vi "oooooldand_upload.vi"() -> ()   [LabVIEW 2016]
uses:
  <userlib>/LevyLab/Graph Utilities/graph_utilities.lvclass
  <userlib>/LevyLab/LV to ITX/Data/Data.lvclass
  <userlib>/LevyLab/postgreSQL-timescaleDB/Data.S3/Data.S3.lvclass
  <userlib>/LevyLab/postgreSQL-timescaleDB/Data.PG/Data.PGSQL.lvclass
  <userlib>/LevyLab/Graph Utilities/graph_utilities.lvclass/graph_utilities.ctl
  <userlib>/LevyLab/LV to ITX/Data/Typedefs/File Type--enum.ctl
  <userlib>/LevyLab/LV to ITX/Data/Data.lvclass/Data.ctl
  <userlib>/_OpenG.lib/file/file.llb/File Exists - Scalar__ogtk.vi
  <userlib>/_OpenG.lib/file/file.llb/Build Path - File Names Array__ogtk.vi
  <userlib>/LevyLab/LV to ITX/Macros/Conversion.lvclass
panel:
  out "Intensity Graph":dbl[][](graph)
  out "Notes":string
  out "cache file out":path
  out "Vertical Linecut":cluster{"Array":dbl[], "A x Vector":dbl[]}[](graph) caption="XY Graph"
  out "Horizontal Linecut":cluster{"Array":dbl[], "A x Vector":dbl[]}[](graph) caption="XY Graph"
  in  "# std deviations for\nhistogram width":dbl(slide)=1.4340101522842639 scale=0.0..5.0
  out "Histogram Graph":T1(graph)={"X Values"=[-4.260453721936876e-06, -4.186170219584622e-06, -4.111886717232367e-06, -4.037603214880112e-06, -3.9633197125278575e-06, -3.889036210175604e-06, -3.814752707823349e-06, -3.7404692054710943e-06, -3.6661857031188396e-06, -3.591902200766585e-06, -3.5176186984143303e-06, -3.4433351960620756e-06, -3.369051693709821e-06, -3.294768191357566e-06, -3.2204846890053115e-06, -3.1462011866530572e-06, -3.0719176843008025e-06, -2.9976341819485483e-06, -2.9233506795962936e-06, -2.849067177244039e-06, -2.774783674891784e-06, -2.7005001725395295e-06, -2.626216670187275e-06, -2.55193316783502e-06, -2.4776496654827654e-06, -2.4033661631305107e-06, -2.3290826607782565e-06, -2.2547991584260018e-06, -2.180515656073747e-06, -2.106232153721493e-06, -2.031948651369238e-06, -1.9576651490169834e-06, -1.8833816466647288e-06, -1.809098144312474e-06, -1.7348146419602196e-06, -1.6605311396079651e-06, -1.5862476372557104e-06, -1.5119641349034557e-06, -1.437680632551201e-06, -1.3633971301989466e-06, -1.289113627846692e-06, -1.2148301254944374e-06, -1.1405466231421827e-06, -1.066263120789928e-06, -9.919796184376733e-07, -9.176961160854188e-07, -8.434126137331644e-07, -7.691291113809097e-07, -6.94845609028655e-07, -6.205621066764003e-07, -5.462786043241458e-07, -4.7199510197189133e-07, -3.9771159961963664e-07, -3.2342809726738195e-07, -2.4914459491512726e-07, -1.7486109256287257e-07, -1.0057759021061788e-07, -2.6294087858363186e-08, 4.798941449389108e-08, 1.2227291684614535e-07, 1.9655641919840004e-07, 2.7083992155065473e-07, 3.451234239029094e-07, 4.194069262551641e-07, 4.936904286074188e-07, 5.679739309596735e-07, 6.422574333119282e-07, 7.165409356641829e-07, 7.908244380164376e-07, 8.651079403686918e-07, 9.393914427209461e-07, 1.0136749450732008e-06, 1.0879584474254555e-06, 1.1622419497777102e-06, 1.2365254521299649e-06, 1.3108089544822195e-06, 1.3850924568344742e-06, 1.459375959186729e-06, 1.5336594615389836e-06, 1.6079429638912379e-06, 1.6822264662434922e-06, 1.7565099685957468e-06, 1.8307934709480015e-06, 1.9050769733002562e-06, 1.979360475652511e-06, 2.0536439780047656e-06, 2.1279274803570203e-06, 2.202210982709275e-06, 2.2764944850615297e-06, 2.3507779874137844e-06, 2.4250614897660386e-06, 2.499344992118293e-06, 2.5736284944705476e-06, 2.6479119968228023e-06, 2.722195499175057e-06, 2.7964790015273117e-06, 2.8707625038795664e-06, 2.945046006231821e-06, 3.0193295085840757e-06, 3.09361301093633e-06], "Histogram: h(x)"=[55, 64, 64, 55, 89, 72, 77, 95, 93, 93, 89, 83, 103, 107, 94, 103, 104, 123, 108, 131, 122, 143, 132, 148, 168, 174, 204, 248, 183, 187, 243, 200, 217, 226, 238, 254, 185, 182, 212, 219, 221, 318, 385, 545, 593, 736, 735, 784, 778, 858, 957, 1241, 1705, 2411, 3715, 13259, 21719, 20305, 20447, 22279, 10136, 3576, 2142, 1564, 1112, 936, 844, 776, 734, 696, 601, 535, 390, 337, 334, 301, 271, 341, 294, 279, 254, 216, 170, 148, 122, 140, 100, 114, 127, 147, 102, 114, 129, 135, 110, 105, 90, 91, 93, 96]}
  in  "menu select":T2(tab)
  in  "Populate Local Tree":bool
  in  "Local Tree":string(tree)
  in  "S3 Connect":bool
  in  "local data directory":path=path "C:/bigdata/PPMS2/SA03008N.20190801/031_sg1_-1'1''5m_3AC=500m_bg=-14" caption="Path"
  in  "Load":bool
  in  "Regen Cache":bool
  out "generating cache":bool
  out "reading cache":bool
  out "cache found":bool
  in  "Visualize":bool
  out "itx load (ms)":u32
  out "cache load (ms)":u32
  out "generate cache (ms)":u32
  out "data dimensions":i32[](array[numeric])
  in  "Remote Tree":string(tree)
  in  "Button":bool
  in  "object path for AWS download":string
  in  "Download\nfrom AWS":bool
  in  "Upload\nto AWS":bool
  out "TDMS file exists on AWS":bool
  out "downloaded file":path
  in  "aws bucket":string="levylab-data"
  in  "path to aws credentials":path=path "C:/Users/phil/.aws/credentials"
  in  "connection info":T3
  in  "Add Op":bool
  in  "Operations List":i32(listbox)
  in  "update":bool
  out "updating":bool
  in  "auto\nupdate":bool
  in  "trash can":i32(listbox)
  in  "OK":bool
  # "4"
  # "7"
  # "10"
  # "12"
  # "14"
  # "Settings"
  # "17"
  # "(e.g. SA03008N.20190801)"
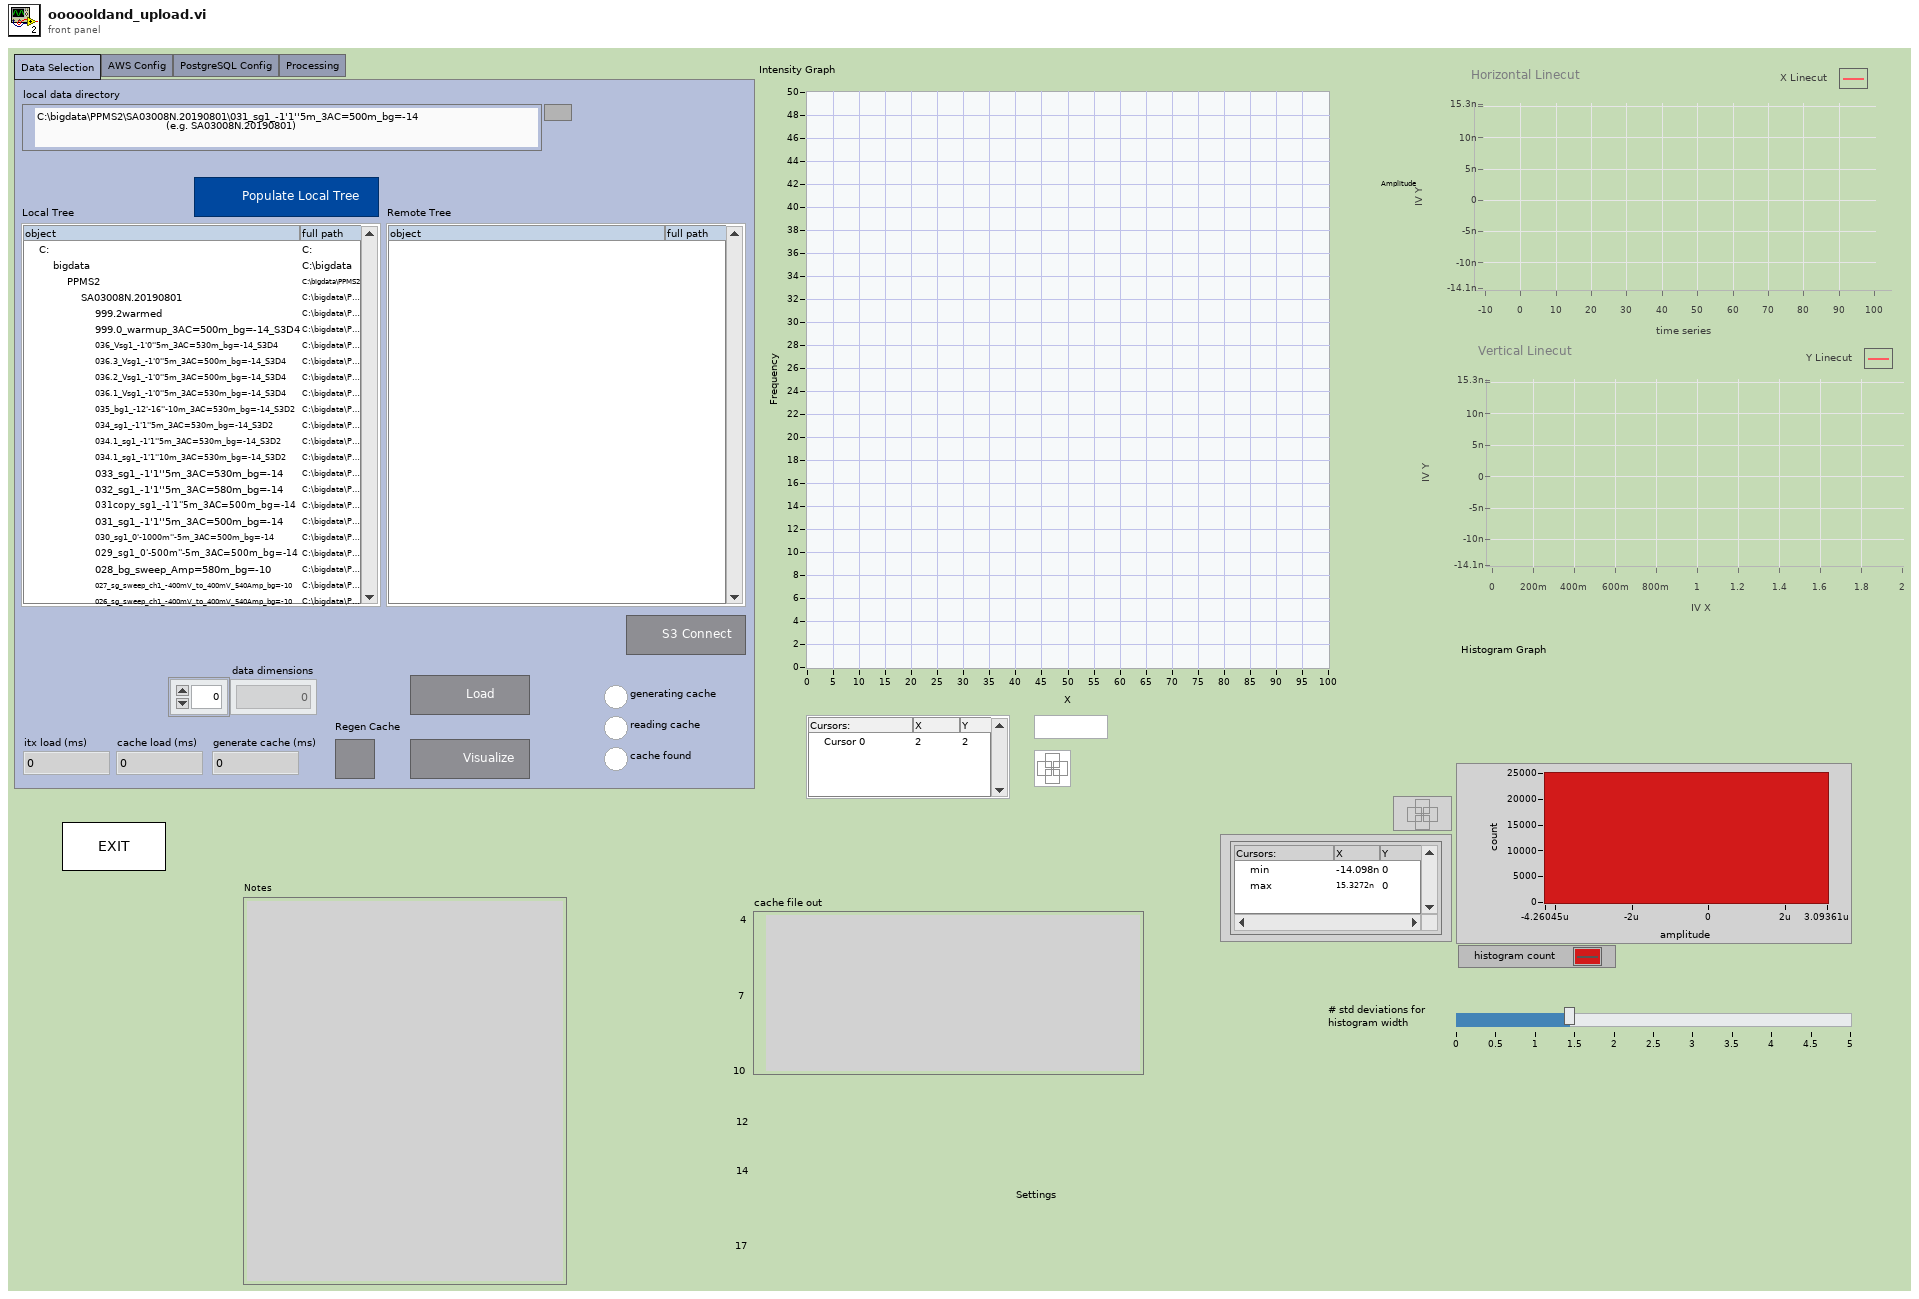
[diagram p1: front panel]
types:
  T1 = cluster{"X Values":dbl[], "Histogram: h(x)":i32[]}
  T2 = enum32{"Data Selection", "AWS Config", "PostgreSQL Config", "Processing"}
  T3 = cluster{"host":string, "port":string, "user":string, "dbname":string, "password":string}
  T4 = enum32{"Invalid", "Standard", "Closed", "Hidden", "Minimized", "Maximized"}
  T5 = enum32{"invalid app kind", "Development System", "Run Time System", "Student Edition", "Embedded LabVIEW", "Evaluation", "Custom"}
  T6 = typedef "Data.lvclass/File Type--enum.ctl" = enum16{"DAT", "ITX", "TDMS", "VI"}
  T7 = typedef "Dictionary Object RefNum__ogtk.ctl" = refnum<k1>
  T8 = cluster{"Core":cluster{"Current VI Reference":refnum<vi>, "Close Panel on Exit?":bool}, "active XY data":cluster{"All expt data":dbl[], "All expt data":dbl[]}[], "local data directory":path, "Data Save":refnum<class "Data.lvclass">, "graphs":refnum<class "graph_utilities.lvclass">[], "dictionary out":T7, "Operations List":refnum<vi>, "operations performed":string[], "Histogram Data":cluster{"X Values":dbl[], "Histogram: h(x)":i32[]}, "Histogram Graph":refnum<vi>, "wavenames":string[], "Data.S3":refnum<class "Data.S3.lvclass">, "data dimensions":i32[], "Data.PG in":refnum<class "Data.PGSQL.lvclass">}
  T9 = cluster{"All expt data":dbl[], "All expt data":dbl[]}[]
  T10 = cluster{"Current VI Reference":refnum<vi>, "Close Panel on Exit?":bool}
  T11 = typedef "Data.lvclass/Dictionary--cluster.ctl" = cluster{"key":string, "value":variant}
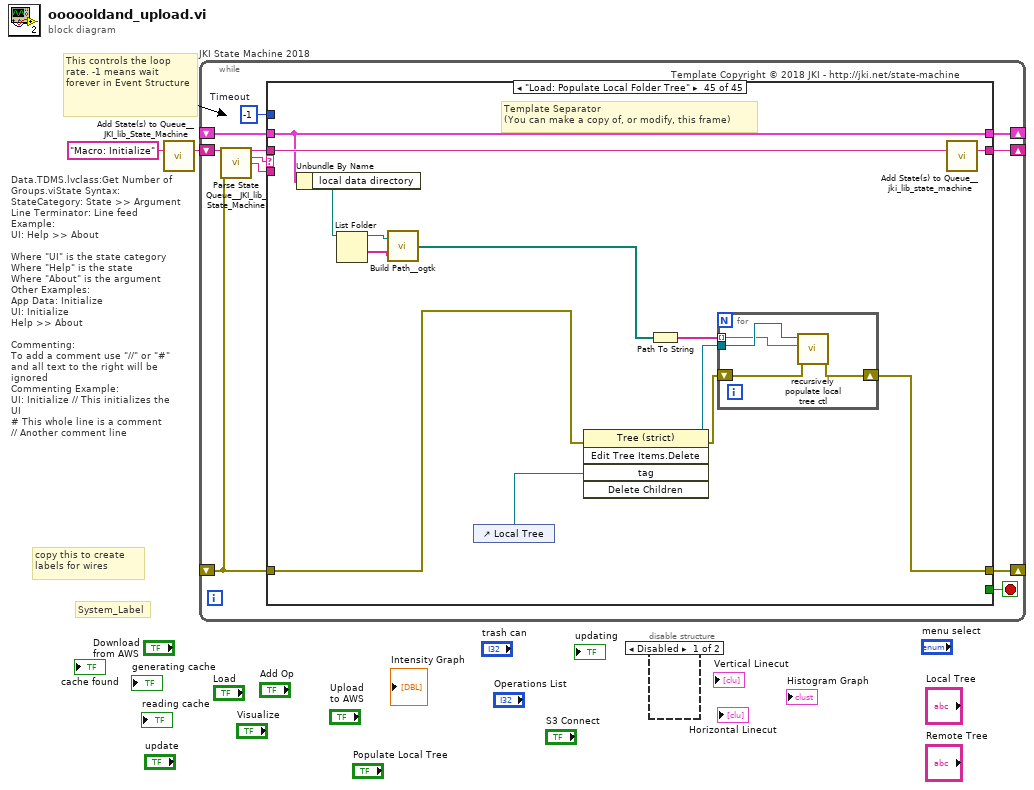
[diagram p0: block diagram]
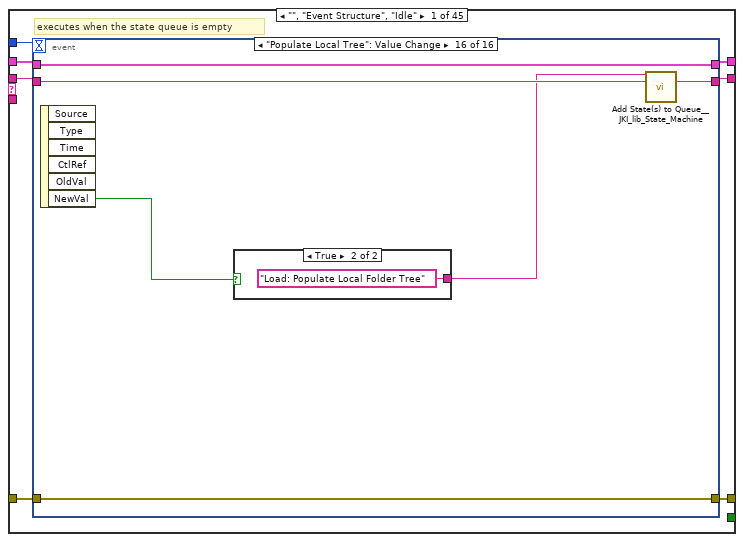
[diagram p3: hidden frame]
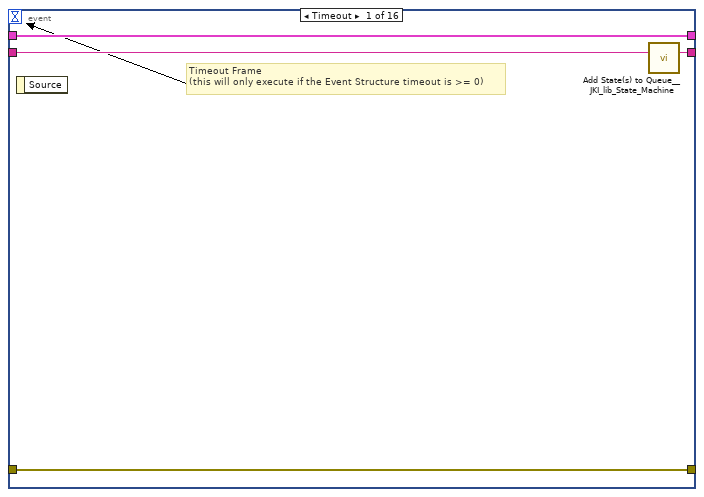
[diagram p4: hidden frame]
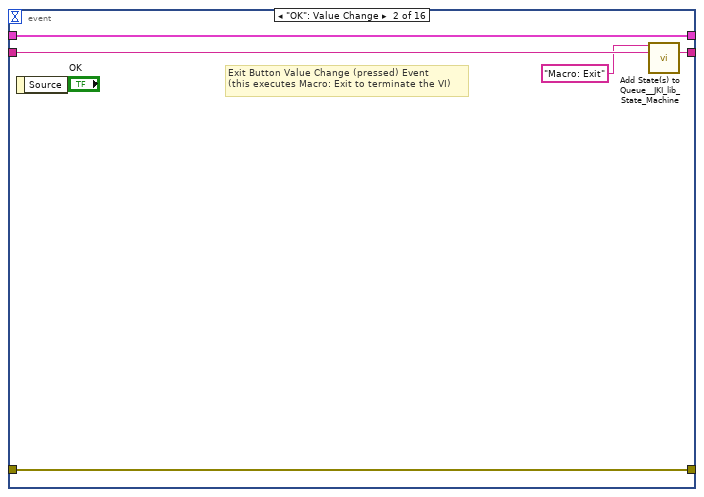
[diagram p5: hidden frame]
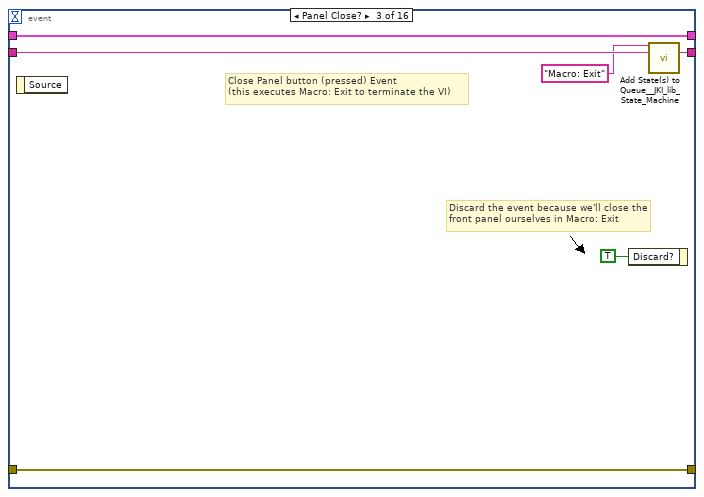
[diagram p6: hidden frame]
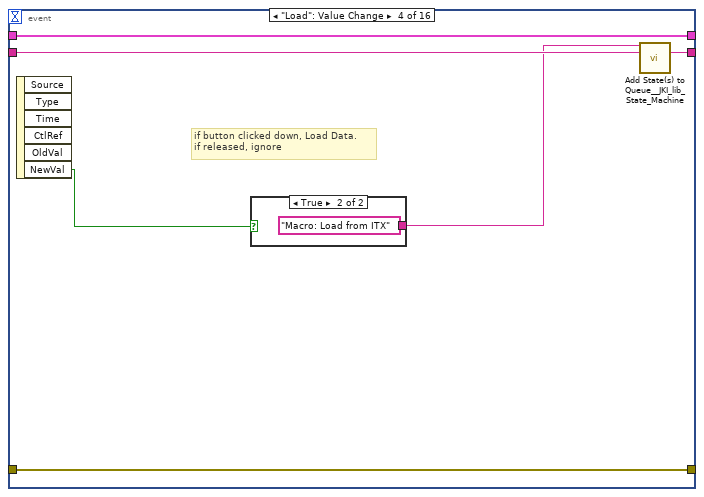
[diagram p7: hidden frame]
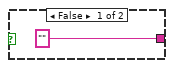
[diagram p8: hidden frame]
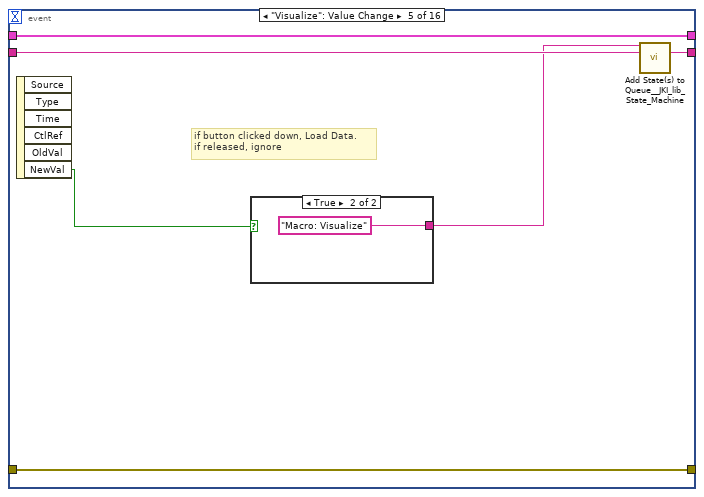
[diagram p9: hidden frame]
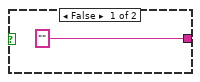
[diagram p10: hidden frame]
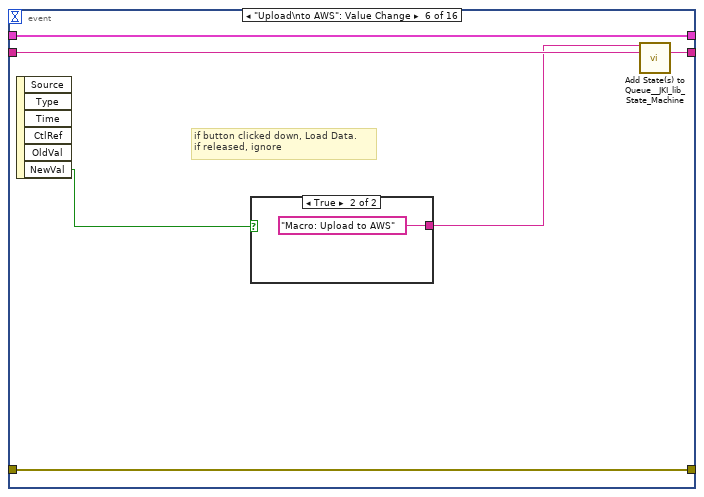
[diagram p11: hidden frame]
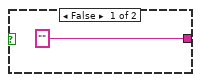
[diagram p12: hidden frame]
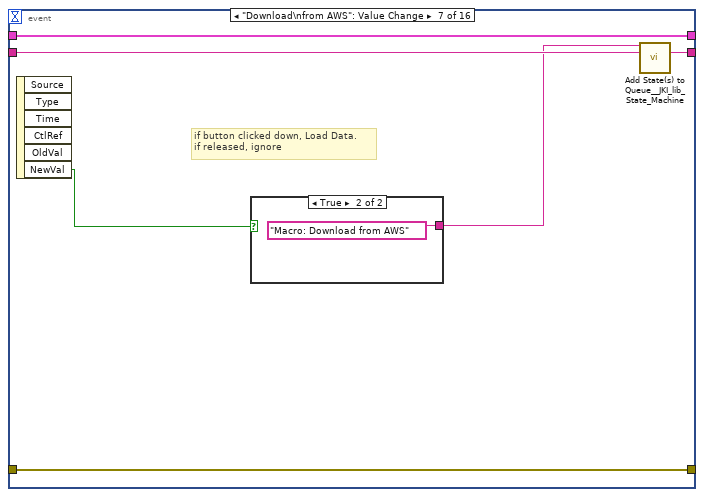
[diagram p13: hidden frame]
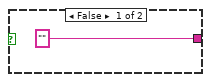
[diagram p14: hidden frame]
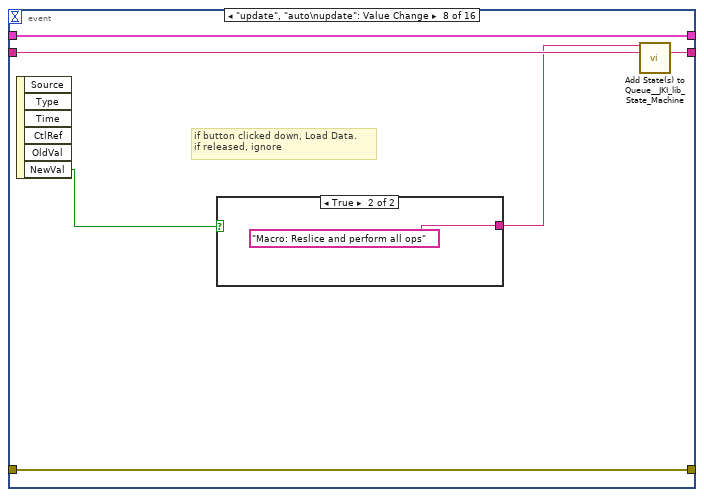
[diagram p15: hidden frame]
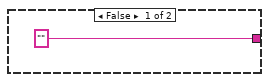
[diagram p16: hidden frame]
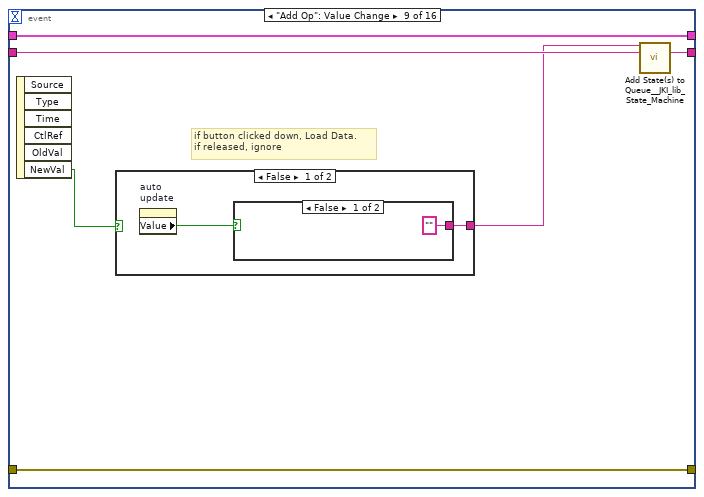
[diagram p17: hidden frame]
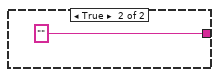
[diagram p18: hidden frame]
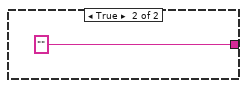
[diagram p19: hidden frame]
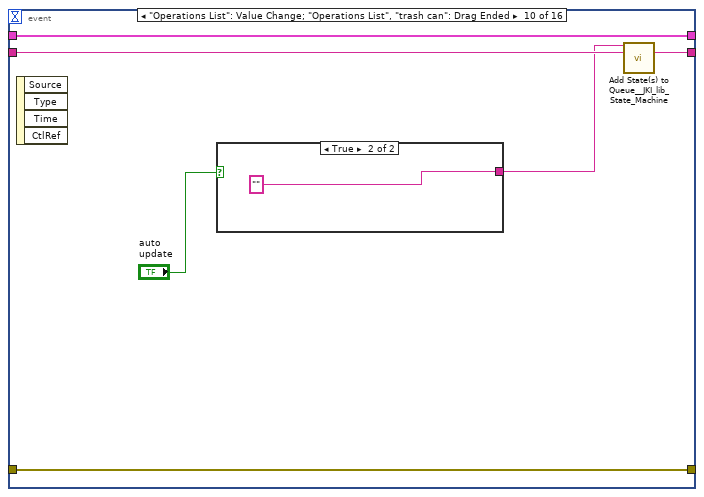
[diagram p20: hidden frame]
diagram:
  # "Data.TDMS.lvclass:Get Number of Groups.viState Syntax:\nStateCategory: State >> Argument\nLine Terminator: Line feed\nExample:\nUI: Help >> About\n\nWhere \"UI\" is the state category\nWhere \"Help\" is the state\nWhere \"About\" is the argument\nOther Examples:\nApp Data: Initialize\nUI: Initialize\nHelp >> About\n\nCommenting:\nTo add a comment use \"//\" or \"#\" and all text to the right will be ignored\nCommenting Example:\nUI: Initialize // This initializes the UI\n# This whole line is a comment\n// Another comment line"
  # "copy this to create labels for wires"
  # "This controls the loop rate. -1 means wait forever in Event Structure"
  # "System_Label"
  n1 = call <vilib>:"Add State(s) to Queue__JKI_lib_State_Machine.vi"("State(s) in (\"\")"="Macro: Initialize") -> ("States Out"=w2:string)  [unwired: 14 in]
  n2 = while "JKI State Machine 2018" {
    shift-right: [w6] -> _
    shift-left: _ -> [w3]
    shift-right: [w9] -> _
    shift-left: _ -> [w4]
    shift-right: [w8] -> _
    shift-left: w2 -> [w10]
    stop <- w7 stop-if-true
    w5 = -1  # Timeout
    # "Template Copyright © 2018 JKI - http://jki.net/state-machine"
    n3 = call <vilib>:"Parse State Queue__JKI_lib_State_Machine.vi"("State Queue"=w10, "Error In (no error)"=w4) -> ("Remaining States"=w12:string, "Current State"=w13:string, "Arguments"=w11:string)  [unwired: 11 in]
    n4 = case shown="\"Load: Populate Local Folder Tree\"" w13 {
      selector: w13 -> [_ _ w137 _ _ _ _ _ _ _ _ _ _ _ _ _ _ _ _ _ _ _ _ _ _ _ _ _ _ _ _ _ _ _ _ _ _ _ _ _ _ _ _ _ _]
      tunnel: w12 -> [w20 w136 w141 w160 w166 w171 w175 w196 w220 w226 w230 w234 w240 w251 w320 w325 w330 w335 w340 w345 w350 w355 w365 w369 w373 w377 w381 w394 w408 w431 w454 w458 w463 w467 w471 w484 w499 w517 w531 w535 w556 w585 w618 w630 w646]
      tunnel: w11 -> [_ _ _ _ _ _ _ _ _ _ _ _ w235 w245 _ _ _ _ _ _ _ _ _ _ _ _ _ _ _ _ _ _ _ _ _ _ _ _ _ _ _ _ _ _ _]
      tunnel: w3 -> [w18 w133 w139 w153 w163 w169 w172 _ w208 w221 w227 w232 w238 w247 w317 w322 w327 w332 w337 w342 w347 w352 w362 w366 w370 w374 w378 w392 w397 w410 w452 w455 w460 w464 w468 w476 w495 w515 w529 w532 w537 w577 w611 w627 w634]
      tunnel: [w17 w134 w143 w157 errorcluster {"status"=FALSE, "code"=0, "source"=""} ("error out") w168 w173 w189 w214 w222 w228 w231 w236 w248 w318 w323 w326 w331 w336 w341 w346 w351 w363 w367 w371 w375 w379 w387 w398 w421 w447 w456 w461 w465 w469 w474 w487 w508 w521 w533 w546 w580 w613 w622 w641] -> w9
      tunnel: w4 -> [w16 w134 w142 w157 w162 w168 w173 w190 w198 w223 w228 w231 w237 w249 w318 w323 w326 w331 w336 w341 w346 w351 w363 w367 w371 w375 w379 w388 w399 w415 w441 w456 w461 w465 w469 w477 w496 w509 w522 w533 w548 w579 w615 w625 w636]
      tunnel: [w19 w135 w140 w159 w165 w170 w174 w195 w219 w225 w229 w233 w239 w250 w319 w324 w329 w334 w339 w344 w349 w354 w364 w368 w372 w376 w380 w393 w407 w430 w453 w457 w462 w466 w470 w483 w498 w516 w530 w534 w555 w584 w617 w629 w645] -> w8
      tunnel: [_ _ _ _ _ TRUE _ _ _ _ _ _ _ _ _ _ _ _ _ _ _ _ _ _ _ _ _ _ _ _ _ _ _ _ _ _ _ _ _ _ _ _ _ _ _] -> w7
      tunnel: [w15 w133 w139 w158 w163 w169 w172 w194 w218 w221 w227 w232 w238 w247 w317 w322 w327 w332 w337 w342 w347 w352 w362 w366 w370 w374 w378 w392 w396 w411 w452 w455 w460 w464 w468 w476 w495 w515 w529 w532 w537 w577 w610 w628 w634] -> w6
      tunnel: w5 -> [w14 _ _ _ _ _ _ _ _ _ _ _ _ _ _ _ _ _ _ _ _ _ _ _ _ _ _ _ _ _ _ _ _ _ _ _ _ _ _ _ _ _ _ _ _]
      frame "", "Event Structure", "Idle" {
        # "executes when the state queue is empty"
        n5 = event shown="[15] \"Populate Local Tree\": Value Change" {
          selector: _ -> [_ _ _ _ _ _ _ _ _ _ _ _ _ _ _ _]
          dyn-events: _ -> [_ _ _ _ _ _ _ _ _ _ _ _ _ _ _ _]
          timeout: w14 -> [_ _ _ _ _ _ _ _ _ _ _ _ _ _ _ _]
          tunnel: w20 -> [w24 w29 w35 w38 w46 w54 w62 w70 w78 w91 w96 w104 w109 w113 w119 w127]
          tunnel: [w23 w28 w34 w39 w47 w55 w63 w71 w79 w90 w97 w103 w108 w114 w120 w128] -> w19
          tunnel: w18 -> [w21 w26 w32 w41 w49 w57 w65 w73 w81 w87 w100 w106 w111 w116 w122 w130]
          tunnel: [w22 w27 w33 w40 w48 w56 w64 w72 w80 w92 w101 w105 w110 w115 w121 w129] -> w17
          tunnel: w16 -> [w22 w27 w33 w40 w48 w56 w64 w72 w80 w92 w101 w105 w110 w115 w121 w129]
          tunnel: [w21 w26 w32 w41 w49 w57 w65 w73 w81 w87 w99 w106 w111 w116 w122 w130] -> w15
          event Timeout {
            # "Timeout Frame\n(this will only execute if the Event Structure timeout is >= 0)"
            n6 = event-data() -> ()  [unwired: 1 in, 1 out]
            n7 = call <vilib>:"Add State(s) to Queue__JKI_lib_State_Machine.vi"("State(s) in (\"\")"=w24) -> ("States Out"=w23:string)  [unwired: 14 in]
          }
          event "OK": Value Change {
            # "Exit Button Value Change (pressed) Event\n(this executes Macro: Exit to terminate the VI)"
            n8 = event-data() -> ()  [unwired: 1 in, 1 out]
            n9 = call <vilib>:"Add State(s) to Queue__JKI_lib_State_Machine.vi"("State(s) in Front (\"\")"="Macro: Exit", "State(s) in (\"\")"=w29) -> ("States Out"=w28:string)  [unwired: 13 in]
          }
          event Panel Close? {
            # "Discard the event because we'll close the front panel ourselves in Macro: Exit"
            # "Close Panel button (pressed) Event\n(this executes Macro: Exit to terminate the VI)"
            n10 = event-data() -> ()  [unwired: 1 in, 1 out]
            n11 = event-data("Discard?"=TRUE) -> ()  [unwired: 1 in, 1 out]
            n12 = call <vilib>:"Add State(s) to Queue__JKI_lib_State_Machine.vi"("State(s) in Front (\"\")"="Macro: Exit", "State(s) in (\"\")"=w35) -> ("States Out"=w34:string)  [unwired: 13 in]
          }
          event "Load": Value Change {
            # "if button clicked down, Load Data.\nif released, ignore"
            n13 = event-data() -> ("NewVal"=w37:bool)  [unwired: 1 in, 5 out]
            n14 = case shown="True" w37 {
              tunnel: ["" "Macro: Load from ITX"] -> w36
              frame False {
              }
              frame True {
              }
            }
            n15 = call <vilib>:"Add State(s) to Queue__JKI_lib_State_Machine.vi"("State(s) in Front (\"\")"=w36, "State(s) in (\"\")"=w38) -> ("States Out"=w39:string)  [unwired: 13 in]
          }
          event "Visualize": Value Change {
            # "if button clicked down, Load Data.\nif released, ignore"
            n16 = event-data() -> ("NewVal"=w45:bool)  [unwired: 1 in, 5 out]
            n17 = case shown="True" w45 {
              tunnel: ["" "Macro: Visualize"] -> w44
              frame False {
              }
              frame True {
              }
            }
            n18 = call <vilib>:"Add State(s) to Queue__JKI_lib_State_Machine.vi"("State(s) in Front (\"\")"=w44, "State(s) in (\"\")"=w46) -> ("States Out"=w47:string)  [unwired: 13 in]
          }
          event "Upload\nto AWS": Value Change {
            # "if button clicked down, Load Data.\nif released, ignore"
            n19 = event-data() -> ("NewVal"=w53:bool)  [unwired: 1 in, 5 out]
            n20 = case shown="True" w53 {
              tunnel: ["" "Macro: Upload to AWS"] -> w52
              frame False {
              }
              frame True {
              }
            }
            n21 = call <vilib>:"Add State(s) to Queue__JKI_lib_State_Machine.vi"("State(s) in Front (\"\")"=w52, "State(s) in (\"\")"=w54) -> ("States Out"=w55:string)  [unwired: 13 in]
          }
          event "Download\nfrom AWS": Value Change {
            # "if button clicked down, Load Data.\nif released, ignore"
            n22 = event-data() -> ("NewVal"=w61:bool)  [unwired: 1 in, 5 out]
            n23 = case shown="True" w61 {
              tunnel: ["" "Macro: Download from AWS"] -> w60
              frame False {
              }
              frame True {
              }
            }
            n24 = call <vilib>:"Add State(s) to Queue__JKI_lib_State_Machine.vi"("State(s) in Front (\"\")"=w60, "State(s) in (\"\")"=w62) -> ("States Out"=w63:string)  [unwired: 13 in]
          }
          event "update", "auto\nupdate": Value Change {
            # "if button clicked down, Load Data.\nif released, ignore"
            n25 = event-data() -> ("NewVal"=w69:bool)  [unwired: 1 in, 5 out]
            n26 = case shown="True" w69 {
              tunnel: ["" "Macro: Reslice and perform all ops"] -> w68
              frame False {
              }
              frame True {
              }
            }
            n27 = call <vilib>:"Add State(s) to Queue__JKI_lib_State_Machine.vi"("State(s) in Front (\"\")"=w68, "State(s) in (\"\")"=w70) -> ("States Out"=w71:string)  [unwired: 13 in]
          }
          event "Add Op": Value Change {
            # "if button clicked down, Load Data.\nif released, ignore"
            n28 = event-data() -> ("NewVal"=w77:bool)  [unwired: 1 in, 5 out]
            n29 = case shown="False" w77 {
              tunnel: [w83 ""] -> w76
              frame False {
                n30 = property on="auto\nupdate" class="Bool (strict)"() -> ("Value"=w82:bool)  [unwired: 2 in, 2 out]
                n31 = case shown="False" w82 {
                  tunnel: ["" ""] -> w83
                  frame False {
                  }
                  frame True {
                  }
                }
              }
              frame True {
              }
            }
            n32 = call <vilib>:"Add State(s) to Queue__JKI_lib_State_Machine.vi"("State(s) in Front (\"\")"=w76, "State(s) in (\"\")"=w78) -> ("States Out"=w79:string)  [unwired: 13 in]
          }
          event "Operations List": Value Change; "Operations List", "trash can": Drag Ended {
            n33 = event-data() -> ()  [unwired: 1 in, 4 out]
            n34 = case shown="True" "auto\nupdate" {
              tunnel: ["" ""] -> w89
              frame False {
              }
              frame True {
              }
            }
            n35 = call <vilib>:"Add State(s) to Queue__JKI_lib_State_Machine.vi"("State(s) in Front (\"\")"=w89, "State(s) in (\"\")"=w91) -> ("States Out"=w90:string)  [unwired: 13 in]
          }
          event "local data directory": Value Change {
            # "if button clicked down, Load Data.\nif released, ignore"
            n36 = event-data() -> ("NewVal"=w95:path)  [unwired: 1 in, 5 out]
            n37 = Bundle By Name(cluster=w100, "local data directory"=w95) -> (w99:T8)
            n38 = call <vilib>:"Add State(s) to Queue__JKI_lib_State_Machine.vi"("State(s) in Front (\"\")"="Load: Check for Cache" ("State(s) in Front (\"\")"), "State(s) in (\"\")"=w96) -> ("States Out"=w97:string)  [unwired: 13 in]
          }
          event "Histogram Graph": Cursor Move {
            n39 = event-data() -> ()  [unwired: 1 in, 9 out]
            n40 = call <vilib>:"Add State(s) to Queue__JKI_lib_State_Machine.vi"("State(s) in Front (\"\")"="Visualize: Update Z from Histogram" ("State(s) in Front (\"\")"), "State(s) in (\"\")"=w104) -> ("States Out"=w103:string)  [unwired: 13 in]
          }
          event "# std deviations for\nhistogram width": Value Change {
            n41 = event-data() -> ()  [unwired: 1 in, 6 out]
            n42 = call <vilib>:"Add State(s) to Queue__JKI_lib_State_Machine.vi"("State(s) in Front (\"\")"="Visualize: Calculate Histogram\nVisualize: Update Z from Histogram" ("State(s) in Front (\"\")"), "State(s) in (\"\")"=w109) -> ("States Out"=w108:string)  [unwired: 13 in]
          }
          event "Intensity Graph": Cursor Move {
            n43 = event-data() -> ()  [unwired: 1 in, 9 out]
            n44 = call <vilib>:"Add State(s) to Queue__JKI_lib_State_Machine.vi"("State(s) in Front (\"\")"="Visualize: Line Cuts" ("State(s) in Front (\"\")"), "State(s) in (\"\")"=w113) -> ("States Out"=w114:string)  [unwired: 13 in]
          }
          event "S3 Connect": Value Change {
            n45 = event-data() -> ("NewVal"=w117:bool)  [unwired: 1 in, 5 out]
            n46 = case shown="True" w117 {
              tunnel: ["" "Macro: Connect to AWS S3" ("State(s) in Front (\"\")")] -> w118
              frame False {
              }
              frame True {
              }
            }
            n47 = call <vilib>:"Add State(s) to Queue__JKI_lib_State_Machine.vi"("State(s) in Front (\"\")"=w118, "State(s) in (\"\")"=w119) -> ("States Out"=w120:string)  [unwired: 13 in]
          }
          event "Populate Local Tree": Value Change {
            n48 = event-data() -> ("NewVal"=w125:bool)  [unwired: 1 in, 5 out]
            n49 = case shown="True" w125 {
              tunnel: ["" "Load: Populate Local Folder Tree" ("State(s) in Front (\"\")")] -> w126
              frame False {
              }
              frame True {
              }
            }
            n50 = call <vilib>:"Add State(s) to Queue__JKI_lib_State_Machine.vi"("State(s) in Front (\"\")"=w126, "State(s) in (\"\")"=w127) -> ("States Out"=w128:string)  [unwired: 13 in]
          }
        }
      }
      frame "---------- Core ----------" {
        # "Do not put any code in this frame.\n(it is a separator no-op)"
        n51 = call <vilib>:"Add State(s) to Queue__jki_lib_state_machine.vi"("State(s) in (\"\")"=w136) -> ("States Out"=w135:string)  [unwired: 14 in]
      }
      frame Default {
        w146 = 42 items=["No error", "Argument error", "Memory is full", "Out of zone", "End of file", "File already open", "Generic file I/O error", "File not found", "File permission error", "Disk is full", "Duplicate path", "Too many files open", "System feature not enabled", "Resource file not found", "Cannot add resource", "Resource not found", "Image not found", "Image memory error", "Pen does not exist", "Config type invalid", "Config token not found", "Config parse error", "Config memory error", "Bad external code format", "Bad external code offset", "External code not present", "Null window", "Destroy window error", "Null menu", "Print aborted", "Bad print record", "Print driver error", "Windows error during printing", "Memory error during printing", "Print dialog error", "Generic print error", "Invalid device refnum", "Device not found", "Device parameter error", "Device unit error", "Cannot open device", "Device call aborted", "Generic error", "Cancelled by user", "Object ID too low", "Object ID too high", "Object not in heap", "Unknown heap", "Unknown object (invalid DefProc)", "Unknown object (DefProc not in table)", "Message out of range", "Invalid (null) method", "Unknown message", "Manager call not supported", "Bad address", "Network operation in progress", "Network operation timed out", "Connection is busy", "Network attribute not supported", "Network error", "Address in use", "System out of memory", "Connection aborted", "Connection refused", "Not connected", "Already connected", "Connection closed", "Initialization error (interapplication manager)", "Bad occurrence", "Wait on unbound occurrence handler", "Occurrence queue overflow", "Datalog type conflict", "Unused", "Unrecognized type (interapplication manager)", "Memory corrupt", "Failed to make temporary DLL", "Old CIN version", "Drag socket not found", "Failed to load drop-object", "Failed to register OLE object", "Failed to release OLE object", "Format specifier type mismatch", "Unknown format specifier", "Too few format specifiers", "Too many format specifiers", "Scan failed", "Newer CIN version", "Error converting to variant", "Runtime menu error", "Password tampered", "Variant attribute not found", "Incompatible variant data type", "Event data is not available", "Event Store is not present", "Occurrence is not found", "Event Queue is not created", "Event info is not available", "Refnum passed is NULL", "Error retrieving Class GUID", "Error retrieving CoClass GUID", "Error retrieving TypeLib GUID.", "Bad built application magic bytes.", "Specific driver is different from the specific driver associated with the Logical Name.", "There is no session opened to the class driver.", "Max Error", "MAX - Error with config objects", "MAX - Error loading configuration", "MAX - Group not supported"]
        # "Current State"
        # "Do not delete, rename, or modify this frame.\n(this is used to capture unhandled states and typos)"
        # "Handle mistyped state name (developer tool)"
        n52 = Format Into String(format string="Software Exception: Unhandled State \"%s\"." ("message"), error in=w142, w137) -> (resulting string=w145:string, error out=w144:errorcluster)  [unwired: 1 in]
        n53 = call <vilib>:"Error Cluster From Error Code.vi"("show call chain? (False)"=TRUE, "error in (no error)"=w144, "error message (\"\")"=w145, "error code (0)"=w146) -> ("error out"=w143:errorcluster)  [unwired: 5 in]
        n54 = call <vilib>:"Add State(s) to Queue__jki_lib_state_machine.vi"("State(s) in (\"\")"=w141) -> ("States Out"=w140:string)  [unwired: 14 in]
      }
      frame "Initialize Core Data" {
        # "Do not delete, rename, or modify this frame.\n(this is used to determine panel behavior on exit)"
        # "originally closed?"
        # "exe?"
        # "If panel starts closed or is an EXE, then close it when we exit"
        n55 = property class="VI"() -> ("FP.State"=w150:T4)  [unwired: 2 in, 2 out]
        n56 = property class="App"() -> ("App.Kind"=w156:T5)  [unwired: 2 in, 2 out]
        n57 = control-ref of="Current VI Reference"() -> (w151:refnum<vi>)
        n58 = Equal?(x=w150, y=T4."Closed" ("Front Panel Window:State")) -> (x = y?=w148:bool)
        n59 = Equal?(x=w156, y=T5."Run Time System" ("Application:Kind")) -> (x = y?=w154:bool)
        n60 = Or(x=w148, y=w154) -> (x .or. y?=w152:bool)
        n61 = Bundle By Name(cluster=w153, "Core.Current VI Reference"=w151, "Core.Close Panel on Exit?"=w152) -> (w158:T8)
        n62 = call <vilib>:"Add State(s) to Queue__jki_lib_state_machine.vi"("State(s) in (\"\")"=w160) -> ("States Out"=w159:string)  [unwired: 14 in]
      }
      frame "Error Handler" {
        # "Unhandled Error -- Display it"
        # "Handle any errors here.\nYou can also output any states to clean-up after errors occur"
        # "Clear error"
        n63 = call <vilib>:"General Error Handler.vi"("error in (no error)"=w162) -> ()  [unwired: 10 in, 5 out]
        n64 = call <vilib>:"Add State(s) to Queue__jki_lib_state_machine.vi"("State(s) in Front (\"\")"="/* Post Error States", "State(s) in (\"\")"=w166) -> ("States Out"=w165:string)  [unwired: 13 in]
      }
      frame "Exit" {
        # "Do not put any code in this frame.\n(No errors that occur here will be handled.)"
        n65 = call <vilib>:"Add State(s) to Queue__jki_lib_state_machine.vi"("State(s) in (\"\")"=w171) -> ("States Out"=w170:string)  [unwired: 14 in]
      }
      frame "---------- Data ----------" {
        # "Do not put any code in this frame.\n(It is a separator no-op. You can make a copy of this frame to create a new Data frame)"
        n66 = call <vilib>:"Add State(s) to Queue__jki_lib_state_machine.vi"("State(s) in (\"\")"=w175) -> ("States Out"=w174:string)  [unwired: 14 in]
      }
      frame "Data: Initialize" {
        w177 = i32[] []  # data dimensions
        w178 = refnum<class "Data.S3.lvclass"> refnum  # Data.S3
        w179 = string[] []  # wavenames
        w183 = T1 {"X Values"=[], "Histogram: h(x)"=[]}  # Histogram Data
        w184 = string[] []  # operations performed
        w186 = T9 []  # active XY data
        w185 = string[] [] ("Strings []")
        w192 = refnum<class "graph_utilities.lvclass">[] []  # graphs
        w193 = T10 {"Current VI Reference"=refnum, "Close Panel on Exit?"=FALSE}  # Core
        # "# groups in tdms\n    (i.e. # original itx files)\n# channels (time, AIN, AON,\n# points per channel\n    (except the channels\n     that only store 1)"
        # "do not delete - used by framework"
        # "Data names and types of shift register data are defined by this bundle."
        # "Initialize the shift-register data, here.\n(data names are defined by what you wire into the bundle function)"
        n67 = call <userlib>:"Dictionary Create__ogtk.vi"("error in (no error)"=w190) -> ("error out"=w189:errorcluster, "dictionary out"=w191:T7)  [unwired: 9 in]
        n68 = control-ref of="Operations List"() -> (w187:refnum<vi>)
        n69 = property on="trash can" class="LstBox (strict)"("Item Names"=w185) -> ()  [unwired: 2 in, 2 out]
        n70 = property class="LstBox (strict)"(reference=w187, "Item Names"=w185) -> (reference out=w188:refnum<vi>)  [unwired: 1 in, 1 out]
        n71 = control-ref of="Histogram Graph"() -> (w182:refnum<vi>)
        n72 = Bundle("Core"=w193, "active XY data"=w186, "local data directory"="local data directory", "Data Save"=refnum<class "Data.lvclass"> refnum, "graphs"=w192, "dictionary out"=w191, "Operations List"=w188, "operations performed"=w184, "Histogram Data"=w183, "Histogram Graph"=w182, "wavenames"=w179, "Data.S3"=w178, "data dimensions"=w177, "Data.PG in"=refnum<class "Data.PGSQL.lvclass"> refnum) -> (w194:T8)  [unwired: 1 in]
        n73 = call <vilib>:"Add State(s) to Queue__jki_lib_state_machine.vi"("State(s) in (\"\")"=w196) -> ("States Out"=w195:string)  [unwired: 14 in]
      }
      frame "Data: Initialize Graph References" {
        # "need to somehow set credentials and bucket"
        n74 = control-ref of="Local Tree"() -> (w201:refnum<vi>)
        n75 = invoke on="Invoke Node" class="Tree (strict)" method="Edit Tree Items.Delete"(reference=w201, error in=w198) -> (error out=w199:errorcluster)  [unwired: 3 in, 4 out]
        n76 = control-ref of="Vertical Linecut"() -> (w211:refnum<vi>)
        n77 = control-ref of="Intensity Graph"() -> (w202:refnum<vi>)
        n78 = Unbundle By Name(w208) -> ("Data.S3"=w207:refnum<class "Data.S3.lvclass">)
        n79 = control-ref of="Remote Tree"() -> (w200:refnum<vi>)
        n80 = control-ref of="Horizontal Linecut"() -> (w212:refnum<vi>)
        n81 = invoke on="Invoke Node" class="Tree (strict)" method="Edit Tree Items.Delete"(reference=w200, error in=w199) -> (error out=w197:errorcluster)  [unwired: 3 in, 4 out]
        n82 = call <userlib>:"Read Credentials from File.vi"("path to aws credentials"="path to aws credentials", "Data.S3"=w207) -> ("Data.S3 out"=w203:refnum<class "Data.S3.lvclass">)  [unwired: 8 in, 1 out]
        n83 = call <userlib>:"Set Bucket.vi"("Bucket name"="aws bucket", "Data.S3"=w203) -> ("Data.S3"=w206:refnum<class "Data.S3.lvclass">)  [unwired: 8 in, 1 out]
        n84 = call <userlib>:"Write Intensity Graph ref.vi"("error in (no error)"=w197, "Intensity Graph (Control)"=w202, "Intensity Graph"=w202) -> ("error out"=w216:errorcluster, "graph_utilities out"=w210:refnum<class "graph_utilities.lvclass">)  [unwired: 7 in]
        n85 = call <userlib>:"Write XY Graph ref.vi"("error in (no error)"=w216, "XY Graph"=w211, "graph_utilities in"=w210) -> ("error out"=w215:errorcluster, "graph_utilities out"=w209:refnum<class "graph_utilities.lvclass">)  [unwired: 7 in]
        n86 = call <userlib>:"Write XY Graph ref.vi"("error in (no error)"=w215, "XY Graph"=w212, "graph_utilities in"=w210) -> ("error out"=w214:errorcluster, "graph_utilities out"=w213:refnum<class "graph_utilities.lvclass">)  [unwired: 7 in]
        n87 = Build Array(w210, w209, w213) -> (w217:refnum<class "graph_utilities.lvclass">[])
        n88 = Bundle By Name(cluster=w208, "graphs"=w217, "Data.S3"=w206) -> (w218:T8)
        n89 = call <vilib>:"Add State(s) to Queue__jki_lib_state_machine.vi"("State(s) in (\"\")"=w220) -> ("States Out"=w219:string)  [unwired: 14 in]
      }
      frame "Data: Cleanup" {
        # "Cleanup any data and references, here.\n(this is called automatically, by the Macro: Exit)"
        n90 = Unbundle By Name(w221) -> ("Core.Current VI Reference"=w224:refnum<vi>)
        n91 = Close Reference(reference=w224, error in (no error)=w223) -> (error out=w222:errorcluster)
        n92 = call <vilib>:"Add State(s) to Queue__jki_lib_state_machine.vi"("State(s) in (\"\")"=w226) -> ("States Out"=w225:string)  [unwired: 14 in]
      }
      frame "---------- UI ----------" {
        # "Do not put any code in this frame.\n(It is a separator no-op. You can make a copy of this frame to create a new UI frame)"
        n93 = call <vilib>:"Add State(s) to Queue__jki_lib_state_machine.vi"("State(s) in (\"\")"=w230) -> ("States Out"=w229:string)  [unwired: 14 in]
      }
      frame "UI: Initialize" {
        # "Initialize the User Interface, here.\n(this is called automatically, by the Macro: Init)"
        n94 = call <vilib>:"Add State(s) to Queue__jki_lib_state_machine.vi"("State(s) in (\"\")"=w234) -> ("States Out"=w233:string)  [unwired: 14 in]
      }
      frame "UI: Cursor Set" {
        # "Argument"
        # "Set and Unset Cursor Busy.\n(Usage: \"UI: Cursor Set >> Busy|Idle\")"
        n95 = case shown="\"Idle\", Default" w235 {
          tunnel: w237 -> [w242 w244]
          tunnel: [w241 w243] -> w236
          frame "Idle", Default {
            n96 = call <vilib>:"Unset Busy.vi"("error in (no error)"=w242) -> ("error out"=w241:errorcluster)  [unwired: 10 in]
          }
          frame "Busy" {
            n97 = call <vilib>:"Set Busy.vi"("error in (no error)"=w244) -> ("error out"=w243:errorcluster)  [unwired: 9 in, 1 out]
          }
        }
        n98 = call <vilib>:"Add State(s) to Queue__jki_lib_state_machine.vi"("State(s) in (\"\")"=w240) -> ("States Out"=w239:string)  [unwired: 14 in]
      }
      frame "UI: Front Panel State" {
        # "Argument"
        # "Set Front Panel Open or Closed\n(Usage: \"UI: Front Panel State >> Open|Close\")"
        n99 = Unbundle By Name(w247) -> ("Core.Current VI Reference"=w246:refnum<vi>)
        n100 = case shown="\"Minimize\", \"Minimized\"" w245 {
          tunnel: w249 -> [w257 w272 w283 w296 w309]
          tunnel: [w259 w273 w285 w298 w311] -> w248
          tunnel: w246 -> [w258 w270 w284 w297 w310]
          frame "Open", "Standard", Default {
            w252 = T4."Standard" ("State")
            n101 = property class="VI"(reference=w258, error in=w257) -> (reference out=w255:refnum<vi>, error out=w256:errorcluster, "FP.State"=w254:T4)
            n102 = Not Equal?(x=w254, y=w252) -> (x != y?=w253:bool)
            n103 = case shown="True" w253 {
              tunnel: [w263 w265] -> w259
              tunnel: w256 -> [w262 w265]
              tunnel: w255 -> [w261 _]
              tunnel: w252 -> [w260 _]
              frame True {
                n104 = invoke class="VI" method="FP.Open"(reference=w261, error in=w262, "Activate"=TRUE, "State"=w260) -> (error out=w263:errorcluster)  [unwired: 1 in, 4 out]
              }
              frame False {
              }
            }
          }
          frame "Close", "Closed" {
            n105 = property class="VI"(reference=w270, error in=w272) -> (reference out=w269:refnum<vi>, error out=w271:errorcluster, "FP.State"=w267:T4)
            n106 = Not Equal?(x=w267, y=T4."Closed" ("Front Panel Window:State")) -> (x != y?=w266:bool)
            n107 = case shown="True" w266 {
              tunnel: [w274 w277] -> w273
              tunnel: w271 -> [w274 w276]
              tunnel: w269 -> [_ w275]
              frame False {
              }
              frame True {
                n108 = invoke class="VI" method="FP.Close"(reference=w275, error in=w276) -> (error out=w277:errorcluster)  [unwired: 1 in, 2 out]
              }
            }
          }
          frame "Hidden", "Hide" {
            w278 = T4."Hidden" ("State")
            n109 = property class="VI"(reference=w284, error in=w283) -> (reference out=w281:refnum<vi>, error out=w282:errorcluster, "FP.State"=w280:T4)
            n110 = Not Equal?(x=w280, y=w278) -> (x != y?=w279:bool)
            n111 = case shown="True" w279 {
              tunnel: [w289 w290] -> w285
              tunnel: w282 -> [w288 w290]
              tunnel: w281 -> [w287 _]
              tunnel: w278 -> [w286 _]
              frame True {
                n112 = invoke class="VI" method="FP.Open"(reference=w287, error in=w288, "State"=w286) -> (error out=w289:errorcluster)  [unwired: 2 in, 4 out]
              }
              frame False {
              }
            }
          }
          frame "Minimize", "Minimized" {
            w291 = T4."Minimized" ("State")
            n113 = property class="VI"(reference=w297, error in=w296) -> (reference out=w294:refnum<vi>, error out=w295:errorcluster, "FP.State"=w293:T4)
            n114 = Not Equal?(x=w293, y=w291) -> (x != y?=w292:bool)
            n115 = case shown="True" w292 {
              tunnel: [w302 w303] -> w298
              tunnel: w295 -> [w301 w303]
              tunnel: w294 -> [w300 _]
              tunnel: w291 -> [w299 _]
              frame True {
                n116 = invoke class="VI" method="FP.Open"(reference=w300, error in=w301, "State"=w299) -> (error out=w302:errorcluster)  [unwired: 2 in, 4 out]
              }
              frame False {
              }
            }
          }
          frame "Maximize", "Maximized" {
            w304 = T4."Maximized" ("State")
            n117 = property class="VI"(reference=w310, error in=w309) -> (reference out=w307:refnum<vi>, error out=w308:errorcluster, "FP.State"=w306:T4)
            n118 = Not Equal?(x=w306, y=w304) -> (x != y?=w305:bool)
            n119 = case shown="True" w305 {
              tunnel: [w315 w316] -> w311
              tunnel: w308 -> [w314 w316]
              tunnel: w307 -> [w313 _]
              tunnel: w304 -> [w312 _]
              frame True {
                n120 = invoke class="VI" method="FP.Open"(reference=w313, error in=w314, "State"=w312) -> (error out=w315:errorcluster)  [unwired: 2 in, 4 out]
              }
              frame False {
              }
            }
          }
        }
        n121 = call <vilib>:"Add State(s) to Queue__jki_lib_state_machine.vi"("State(s) in (\"\")"=w251) -> ("States Out"=w250:string)  [unwired: 14 in]
      }
      frame "---------- Macro ----------" {
        # "Do not put any code in this frame.\n(It is a separator no-op. You can make a copy of this frame to create a new Macro frame)"
        n122 = call <vilib>:"Add State(s) to Queue__jki_lib_state_machine.vi"("State(s) in (\"\")"=w320) -> ("States Out"=w319:string)  [unwired: 14 in]
      }
      frame "Macro: Initialize" {
        w321 = "Data: Initialize\nData: Initialize Graph References\nInitialize Core Data\nUI: Initialize\nUI: Front Panel State >> Open\nLoad: Check for Cache"  # Data: Initialize Data: Initialize Graph References Initialize Core Data UI: Initialize UI: Front Panel State >> Open Load: Check for Cache
        # "Initialization Macro\n(This is called once, when the VI starts)"
        n123 = call <vilib>:"Add State(s) to Queue__jki_lib_state_machine.vi"("State(s) in Front (\"\")"=w321, "State(s) in (\"\")"=w325) -> ("States Out"=w324:string)  [unwired: 13 in]
      }
      frame "Macro: Load from ITX" {
        # "Initialization Macro\n(This is called once, when the VI starts)"
        n124 = call <vilib>:"Add State(s) to Queue__jki_lib_state_machine.vi"("State(s) in Front (\"\")"="Load: Load from ITX", "State(s) in (\"\")"=w330) -> ("States Out"=w329:string)  [unwired: 13 in]
      }
      frame "Macro: Connect to AWS S3" {
        # "Initialization Macro\n(This is called once, when the VI starts)"
        n125 = call <vilib>:"Add State(s) to Queue__jki_lib_state_machine.vi"("State(s) in Front (\"\")"="AWS: List Bucket Contents", "State(s) in (\"\")"=w335) -> ("States Out"=w334:string)  [unwired: 13 in]
      }
      frame "Macro: Visualize" {
        # "#TODO: should rename this macro,\nit only needs to be sliced after the slicing indices are changed"
        # "Initialization Macro\n(This is called once, when the VI starts)"
        n126 = call <vilib>:"Add State(s) to Queue__jki_lib_state_machine.vi"("State(s) in Front (\"\")"="Visualize: Plot Live XY to Intensity\nVisualize: Calculate Histogram\nVisualize: Update Z from Histogram\nVisualize: Line Cuts", "State(s) in (\"\")"=w340) -> ("States Out"=w339:string)  [unwired: 13 in]
      }
      frame "Macro: Upload to AWS" {
        # "#TODO: should rename this macro,\nit only needs to be sliced after the slicing indices are changed"
        # "Initialization Macro\n(This is called once, when the VI starts)"
        n127 = call <vilib>:"Add State(s) to Queue__jki_lib_state_machine.vi"("State(s) in Front (\"\")"="AWS: Upload file\nAWS: Check if file exists", "State(s) in (\"\")"=w345) -> ("States Out"=w344:string)  [unwired: 13 in]
      }
      frame "Macro: Download from AWS" {
        # "#TODO: should rename this macro,\nit only needs to be sliced after the slicing indices are changed"
        # "Initialization Macro\n(This is called once, when the VI starts)"
        n128 = call <vilib>:"Add State(s) to Queue__jki_lib_state_machine.vi"("State(s) in Front (\"\")"="AWS: Check if file exists\nAWS: Download file", "State(s) in (\"\")"=w350) -> ("States Out"=w349:string)  [unwired: 13 in]
      }
      frame "Macro: Reslice and perform all ops" {
        # "#TODO: should rename this macro,\nit only needs to be sliced after the slicing indices are changed"
        # "Initialization Macro\n(This is called once, when the VI starts)"
        n129 = call <vilib>:"Add State(s) to Queue__jki_lib_state_machine.vi"("State(s) in Front (\"\")"="Macro: Visualize", "State(s) in (\"\")"=w355) -> ("States Out"=w354:string)  [unwired: 13 in]
      }
      frame "Macro: Exit" {
        # "Exit Macro\n(This is called once, when the VI exits)"
        n130 = Unbundle By Name(w362) -> ("Core.Close Panel on Exit?"=w361:bool)
        n131 = Select(t="UI: Front Panel State >> Close", s=w361, f="") -> (s? t:f=w358:string)
        n132 = call <vilib>:"Add State(s) to Queue__jki_lib_state_machine.vi"("State(s) in (\"\")"=w358, "State(s) at Back (\"\")"="Data: Cleanup\nExit") -> ("States Out"=w356:string)  [unwired: 13 in]
        n133 = call <vilib>:"Add State(s) to Queue__jki_lib_state_machine.vi"("State(s) in Front (\"\")"=w356, "State(s) in (\"\")"=w365) -> ("States Out"=w364:string)  [unwired: 13 in]
      }
      frame "---------- New Category ----------" {
        # "Template Separator\n(You can make a copy of, or modify, this frame)"
        n134 = call <vilib>:"Add State(s) to Queue__jki_lib_state_machine.vi"("State(s) in (\"\")"=w369) -> ("States Out"=w368:string)  [unwired: 14 in]
      }
      frame "New Category: 1" {
        # "Your code here.\n(You can make a copy of, or modify, this frame)"
        n135 = call <vilib>:"Add State(s) to Queue__jki_lib_state_machine.vi"("State(s) in (\"\")"=w373) -> ("States Out"=w372:string)  [unwired: 14 in]
      }
      frame "New Category: 2" {
        # "Your code here.\n(You can make a copy of, or modify, this frame)"
        n136 = call <vilib>:"Add State(s) to Queue__jki_lib_state_machine.vi"("State(s) in (\"\")"=w377) -> ("States Out"=w376:string)  [unwired: 14 in]
      }
      frame "---------- AWS ----------" {
        # "Template Separator\n(You can make a copy of, or modify, this frame)"
        n137 = call <vilib>:"Add State(s) to Queue__jki_lib_state_machine.vi"("State(s) in (\"\")"=w381) -> ("States Out"=w380:string)  [unwired: 14 in]
      }
      frame "AWS: Check if file exists" {
        # "Your code here.\n(You can make a copy of, or modify, this frame)"
        n138 = Unbundle By Name(w392) -> ("local data directory"=w389:path, "Data.S3"=w382:refnum<class "Data.S3.lvclass">)
        n139 = Path To String(path=w389) -> (string=w384:string)
        n140 = call "replace_bad_aws_characters.vi"("name"=w384) -> ("result string"=w383:string)  [unwired: 9 in, 1 out]
        n141 = Concatenate Strings(w383, ".tdms") -> (w390:string)
        n142 = String To Path(string=w390) -> (path=w386:path)
        n143 = call <userlib>:"Verify File.vi"("error in (no error)"=w388, "file to check"=w386, "Data.S3"=w382) -> ("error out"=w387:errorcluster, "found somewhere in prefix"=→"TDMS file exists on AWS":bool)  [unwired: 6 in, 1 out]
        n144 = call <vilib>:"Add State(s) to Queue__jki_lib_state_machine.vi"("State(s) in (\"\")"=w394) -> ("States Out"=w393:string)  [unwired: 14 in]
      }
      frame "AWS: List Bucket Contents" {
        # "Your code here.\n(You can make a copy of, or modify, this frame)"
        n145 = Unbundle By Name(w397) -> ("local data directory"=w404:path, "Data.S3"=w401:refnum<class "Data.S3.lvclass">)
        n146 = Path To String(path=w404) -> (string=w403:string)
        n147 = call "replace_bad_aws_characters.vi"("name"=w403) -> ("result string"=w402:string)  [unwired: 9 in, 1 out]
        n148 = Concatenate Strings(w402, ".tdms") -> (w405:string)
        n149 = control-ref of="Remote Tree"() -> (w400:refnum<vi>)
        n150 = String To Path(string=w405) -> ()  [unwired: 1 out]
        n151 = call <userlib>:"Populate Tree Ctl from Bucket.vi"("error in (no error)"=w399, "Tree Ctl Ref"=w400, "Data.S3"=w401) -> ("error out"=w398:errorcluster, "Data.S3 out"=w395:refnum<class "Data.S3.lvclass">)  [unwired: 4 in, 3 out]
        n152 = Bundle By Name(cluster=w397, "Data.S3"=w395) -> (w396:T8)
        n153 = call <vilib>:"Add State(s) to Queue__jki_lib_state_machine.vi"("State(s) in (\"\")"=w408) -> ("States Out"=w407:string)  [unwired: 14 in]
      }
      frame "AWS: Upload file" {
        w424 = "/"
        # "SA030.."
        # "031_.."
        # "#TODO: put these values in the\nstate wire..."
        # "Template Separator\n(You can make a copy of, or modify, this frame)"
        n154 = Unbundle By Name(w410) -> ("local data directory"=w423:path, "Data.S3"=w412:refnum<class "Data.S3.lvclass">)
        n155 = Path To String(path=w423) -> (string=w429:string)
        n156 = Concatenate Strings(w429, ".tdms") -> (w427:string)
        n157 = String To Path(string=w427) -> (path=w422:path)
        n158 = Strip Path(path=w422) -> (stripped path=w425:path, name=w419:string)
        n159 = Strip Path(path=w425) -> (name=w417:string)  [unwired: 1 out]
        n160 = call "replace_bad_aws_characters.vi"("error in (no error)"=w415, "name"=w419) -> ("error out"=w414:errorcluster, "result string"=w418:string)  [unwired: 8 in]
        n161 = call "replace_bad_aws_characters.vi"("error in (no error)"=w414, "name"=w417) -> ("error out"=w413:errorcluster, "result string"=w416:string)  [unwired: 8 in]
        n162 = call-poly <userlib>:"File Exists__ogtk.vi"("file path"=w422) -> ("exists"=w426:bool)  [unwired: 6 in, 1 out]
        n163 = Concatenate Strings(w424, w416, w424, w418) -> (w420:string)
        n164 = case shown="True" w426 {
          tunnel: w422 -> [_ w436]
          tunnel: w420 -> [_ w439]
          tunnel: w413 -> [w433 w438]
          tunnel: [w433 w437] -> w421
          tunnel: w412 -> [w432 w435]
          tunnel: [w432 w434] -> w409
          frame False {
            n165 = call "Display Message to User"() -> ()  [unwired: 10 in, 2 out]
          }
          frame True {
            n166 = call <userlib>:"Upload File.vi"("error in (no error)"=w438, "Object Path (including file name)"=w439, "file to upload"=w436, "Data.S3"=w435) -> ("error out"=w437:errorcluster, "Data.S3"=w434:refnum<class "Data.S3.lvclass">)  [unwired: 6 in]
          }
        }
        n167 = Bundle By Name(cluster=w410, "Data.S3"=w409) -> (w411:T8)
        n168 = call <vilib>:"Add State(s) to Queue__jki_lib_state_machine.vi"("State(s) in (\"\")"=w431) -> ("States Out"=w430:string)  [unwired: 14 in]
      }
      frame "AWS: Download file" {
        # "#TODO: put these values in the\nstate wire..."
        # "Template Separator\n(You can make a copy of, or modify, this frame)"
        n169 = Unbundle By Name(w452) -> ("local data directory"=w449:path, "Data.S3"=w446:refnum<class "Data.S3.lvclass">)
        n170 = Path To String(path=w449) -> (string=w443:string)
        n171 = call "replace_bad_aws_characters.vi"("error in (no error)"=w441, "name"=w443) -> ("error out"=w440:errorcluster, "result string"=w442:string)  [unwired: 8 in]
        n172 = Concatenate Strings(w442, ".tdms") -> (w450:string)
        n173 = String To Path(string=w450) -> (path=w444:path)
        n174 = call <userlib>:"Download File.vi"("error in (no error)"=w440, "Object Path"="object path for AWS download", "path to store downloaded file"=w444, "Data.S3"=w446) -> ("error out"=w447:errorcluster, "file from jeff"=→"downloaded file":path)  [unwired: 5 in, 1 out]
        n175 = call <vilib>:"Add State(s) to Queue__jki_lib_state_machine.vi"("State(s) in (\"\")"=w454) -> ("States Out"=w453:string)  [unwired: 14 in]
      }
      frame "---------- PostgreSQL ----------" {
        # "Template Separator\n(You can make a copy of, or modify, this frame)"
        n176 = call <vilib>:"Add State(s) to Queue__jki_lib_state_machine.vi"("State(s) in (\"\")"=w458) -> ("States Out"=w457:string)  [unwired: 14 in]
      }
      frame "PostgreSQL: Configure Connection" {
        # "Template Separator\n(You can make a copy of, or modify, this frame)"
        n177 = Unbundle By Name(w460) -> ("Data.PG in"=w459:refnum<class "Data.PGSQL.lvclass">)
        n178 = call <userlib>:"Set Connection Info.vi"("Data.PG in"=w459) -> ()  [unwired: 8 in, 2 out]
        n179 = call <vilib>:"Add State(s) to Queue__jki_lib_state_machine.vi"("State(s) in (\"\")"=w463) -> ("States Out"=w462:string)  [unwired: 14 in]
      }
      frame "PostgreSQL: Upload Data" {
        # "Template Separator\n(You can make a copy of, or modify, this frame)"
        n180 = call <vilib>:"Add State(s) to Queue__jki_lib_state_machine.vi"("State(s) in (\"\")"=w467) -> ("States Out"=w466:string)  [unwired: 14 in]
      }
      frame "---------- Visualize ----------" {
        # "Template Separator\n(You can make a copy of, or modify, this frame)"
        n181 = call <vilib>:"Add State(s) to Queue__jki_lib_state_machine.vi"("State(s) in (\"\")"=w471) -> ("States Out"=w470:string)  [unwired: 14 in]
      }
      frame "Visualize: Plot Live XY to Intensity" {
        # "#TODO: Shouldnt go in here"
        n182 = Unbundle By Name(w476) -> ("graphs"=w480:refnum<class "graph_utilities.lvclass">[], "active XY data"=w479:T9)
        n183 = call "XYs_to_Intensity.vi"("error in (no error)"=w477, "XYs in"=w479) -> ("error out"=w478:errorcluster, "Intensity data (y) out"=w481:dbl[][])  [unwired: 8 in]
        n184 = Index Array(array=w480) -> (element=w482:refnum<class "graph_utilities.lvclass">)  [unwired: 1 in]
        n185 = call <userlib>:"Set Intensity Graph Value.vi"("error in (no error)"=w478, "Value"=w481, "graph_utilities in"=w482) -> ("error out"=w475:errorcluster)  [unwired: 7 in, 1 out]
        n186 = property on="updating" class="Bool (strict)"(error in=w475, "Value"=FALSE ("updating")) -> (error out=w474:errorcluster)  [unwired: 1 in, 1 out]
        n187 = call <vilib>:"Add State(s) to Queue__jki_lib_state_machine.vi"("State(s) in Front (\"\")"="Visualize: Calculate Histogram" ("State(s) in Front (\"\")"), "State(s) in (\"\")"=w484) -> ("States Out"=w483:string)  [unwired: 13 in]
      }
      frame "Visualize: Calculate Histogram" {
        n188 = Unbundle By Name(w495) -> ("Histogram Graph"=w491:refnum<vi>, "active XY data"=w497:T9)
        n189 = call "XYs_to_Intensity.vi"("error in (no error)"=w496, "XYs in"=w497) -> ("error out"=w493:errorcluster, "Intensity data (y) out"=w494:dbl[][])  [unwired: 8 in]
        n190 = call "calculate_histogram.vi"("error in (no error)"=w493, "# std deviations for histogram width (1)"="# std deviations for\nhistogram width", "2D arr Intensity Graph"=w494) -> ("error out"=w490:errorcluster, "Histogram Graph"=w492:T1)  [unwired: 5 in, 2 out]
        n191 = property class="XYGraph (strict)"(reference=w491, error in=w490, "Value"=w492) -> (reference out=w489:refnum<vi>, error out=w488:errorcluster)
        n192 = call "adjust_histogram_cursor.vi"("error in (no error)"=w488, "lock to bin edges"=TRUE, "histogram reference"=w489) -> ("error out"=w487:errorcluster)  [unwired: 8 in]
        n193 = call <vilib>:"Add State(s) to Queue__jki_lib_state_machine.vi"("State(s) in (\"\")"=w499) -> ("States Out"=w498:string)  [unwired: 14 in]
      }
      frame "Visualize: Update Z from Histogram" {
        # "#TODO: adjust line cut scales\nhere also"
        n194 = Unbundle By Name(w515) -> ("graphs"=w511:refnum<class "graph_utilities.lvclass">[], "Histogram Graph"=w512:refnum<vi>)
        n195 = property on="Property Node" class="XYGraph (strict)"(reference=w512, error in=w509, "Active Cursor"=u32 0, "Active Cursor"=u32 1) -> (error out=w504:errorcluster, "Cursor.Cursor X"=w503:dbl, "Cursor.Cursor X"=w502:dbl)  [unwired: 1 out]
        n196 = control-ref of="Horizontal Linecut"() -> (w501:refnum<vi>)
        n197 = control-ref of="Vertical Linecut"() -> (w500:refnum<vi>)
        n198 = disable-structure shown="Enabled" {
          disable-tunnel: w511 -> [w518 _]
          disable-tunnel: [_ w519] -> w510
          frame Disabled {
            # "Should have a graphutils\nvi for Z range setting here"
            n199 = Index Array(array=w518) -> ()  [unwired: 1 in, 1 out]
          }
          frame Enabled {
            n200 = control-ref of="Intensity Graph"() -> (w519:refnum<vi>)
          }
        }
        n201 = property on="Property Node" class="IntGraph (strict)"(reference=w510, error in=w504, "ZScale.Minimum"=w503, "ZScale.Maximum"=w502) -> (error out=w507:errorcluster)  [unwired: 1 out]
        n202 = property on="Property Node" class="XYGraph (strict)"(reference=w501, error in=w504, "YScale.Minimum"=w503, "YScale.Maximum"=w502) -> (error out=w506:errorcluster)  [unwired: 1 out]
        n203 = property on="Property Node" class="XYGraph (strict)"(reference=w500, error in=w504, "YScale.Minimum"=w503, "YScale.Maximum"=w502) -> (error out=w505:errorcluster)  [unwired: 1 out]
        n204 = Merge Errors(w507, w506, w505) -> (w508:errorcluster)
        n205 = call <vilib>:"Add State(s) to Queue__jki_lib_state_machine.vi"("State(s) in (\"\")"=w517) -> ("States Out"=w516:string)  [unwired: 14 in]
      }
      frame "Visualize: Line Cuts" {
        w520 = 42.0 ("width (vertical)")
        n206 = disable-structure shown="Disabled" {
          frame Disabled {
            n207 = call <userlib>:"Linecut Example.vi"() -> ()  [unwired: 12 in]
          }
          frame Enabled {
          }
        }
        n208 = Unbundle By Name(w529) -> ("graphs"=w526:refnum<class "graph_utilities.lvclass">[])
        n209 = Index Array(array=w526, index #1=1 ("index"), index #2=2 ("index")) -> (element #1=w525:refnum<class "graph_utilities.lvclass">, element #2=w524:refnum<class "graph_utilities.lvclass">)
        n210 = call <userlib>:"Intensity Graph Linecut (Vertical).vi"("error in (no error)"=w522, "width (vertical)"=w520, "graph_utilities in"=w525) -> ("error out"=w523:errorcluster)  [unwired: 7 in, 1 out]
        n211 = call <userlib>:"Intensity Graph Linecut (Horizontal).vi"("error in (no error)"=w523, "width (horizontal)"=w520, "graph_utilities in"=w524) -> ("error out"=w521:errorcluster)  [unwired: 7 in, 1 out]
        n212 = call <vilib>:"Add State(s) to Queue__jki_lib_state_machine.vi"("State(s) in (\"\")"=w531) -> ("States Out"=w530:string)  [unwired: 14 in]
      }
      frame "---------- Load ----------" {
        # "Template Separator\n(You can make a copy of, or modify, this frame)"
        n213 = call <vilib>:"Add State(s) to Queue__jki_lib_state_machine.vi"("State(s) in (\"\")"=w535) -> ("States Out"=w534:string)  [unwired: 14 in]
      }
      frame "Load: Generate Cache" {
        # "#TODO: 'to generate or not to generate' logic\nshould probably go in a different frame"
        # "if regen cache or not exist:"
        # "Template Separator\n(You can make a copy of, or modify, this frame)"
        n214 = property on="generating cache" class="Bool (strict)"(error in=w548, "Value"=TRUE ("working")) -> (error out=w541:errorcluster)  [unwired: 1 in, 1 out]
        n215 = call <userlib>:"Tick Count (ms)__ogtk.vi"("error in (no error)"=w541) -> ("error out"=w540:errorcluster, "millisecond timer value"=w543:u32)  [unwired: 9 in]
        n216 = Unbundle By Name(w537) -> ("local data directory"=w549:path)
        n217 = call "check_if_cache_exists.vi"("error in (no error)"=w540, "Experiment Folder"=w549) -> ("error out"=w550:errorcluster, "cache file out"=w536:path, "exists"=w554:bool)  [unwired: 7 in]
        n218 = Not(x=w554) -> (.not. x?=w553:bool)
        n219 = Or(x="Regen Cache", y=w553) -> (x .or. y?=w552:bool)
        n220 = case shown="True" w552 {
          tunnel: w550 -> [w557 w562]
          tunnel: [w557 w558] -> w539
          tunnel: w549 -> [_ w560]
          tunnel: w536 -> [_ _]
          frame False {
          }
          frame True {
            # "expt folder"
            # "unnecessary now for tdms\nunless we want to store in a different location"
            # "replaceorcreate"
            n221 = call "TDMS path from Experiment Folder.vi"("error in (no error)"=w562, "experiment folder"=w560) -> ("error out"=w561:errorcluster)  [unwired: 7 in, 2 out]
            n222 = disable-structure shown="Enabled" {
              disable-tunnel: _ -> [w572 _]
              disable-tunnel: w560 -> [w571 w576]
              disable-tunnel: [w570 _] -> _
              disable-tunnel: [w569 w575] -> w559
              disable-tunnel: [w568 _] -> _
              disable-tunnel: [w567 _] -> _
              disable-tunnel: File_Type--enum."ITX" ("Experiment Folder File Type") -> [_ w574]
              disable-tunnel: w561 -> [w566 w573]
              frame Disabled {
                n223 = call "write_itxFolder_to_cache.vi"("error in (no error)"=w566, "experiment folder (containing itx)"=w571, "cache file path"=w572) -> ("error out"=w569:errorcluster, "notes"=w568:string[], "wave names"=w567:string[], "written cache file out"=w570:path)  [unwired: 5 in]
              }
              frame Enabled {
                n224 = call <userlib>:"Convert Experiment Folder.vi"("error in (no error)"=w573, "Experiment Folder File Type"=w574, "Experiment Folder Path"=w576) -> ("error out"=w575:errorcluster)  [unwired: 8 in]
              }
            }
            n225 = disable-structure shown="Disabled" {
              disable-tunnel: w560 -> [_ _]
              disable-tunnel: w559 -> [w564 w565]
              disable-tunnel: [w564 w565] -> w558
              frame Disabled {
                # "unattached\nmetadata\nto TDMS"
              }
              frame Enabled {
              }
            }
          }
        }
        n226 = call <userlib>:"Tick Count (ms)__ogtk.vi"("error in (no error)"=w539) -> ("error out"=w538:errorcluster, "millisecond timer value"=w544:u32)  [unwired: 9 in]
        n227 = Subtract(x=w544, y=w543) -> (x-y=→"generate cache (ms)":u32)
        n228 = property on="generating cache" class="Bool (strict)"(error in=w538, "Value"=FALSE ("working")) -> (error out=w546:errorcluster)  [unwired: 1 in, 1 out]
        n229 = call <vilib>:"Add State(s) to Queue__jki_lib_state_machine.vi"("State(s) in (\"\")"=w556) -> ("States Out"=w555:string)  [unwired: 14 in]
      }
      frame "Load: Check for Cache" {
        # "#TODO: 'to generate or not to generate' logic\nshould probably go in a different frame"
        # "if regen cache or not exist:"
        # "Template Separator\n(You can make a copy of, or modify, this frame)"
        n230 = Unbundle By Name(w577) -> ("local data directory"=w583:path)  [unwired: 1 out]
        n231 = call "check_if_cache_exists.vi"("error in (no error)"=w579, "Experiment Folder"=w583) -> ("error out"=w578:errorcluster, "cache file out"=→"cache file out":path, "exists"=w581:bool)  [unwired: 7 in]
        n232 = property on="cache found" class="Bool (strict)"(error in=w578, "Value"=w581) -> (error out=w580:errorcluster)  [unwired: 1 in, 1 out]
        n233 = call <vilib>:"Add State(s) to Queue__jki_lib_state_machine.vi"("State(s) in (\"\")"=w585) -> ("States Out"=w584:string)  [unwired: 14 in]
      }
      frame "Load: Load from Cache" {
        # "#TODO: clean up frame with more subvis\nalso this will get messed up if a 'single data\npoint' channel is the first one..."
        # "Template Separator\n(You can make a copy of, or modify, this frame)"
        n234 = property on="reading cache" class="Bool (strict)"(error in=w615, "Value"=TRUE ("read cache")) -> (error out=w606:errorcluster)  [unwired: 1 in, 1 out]
        n235 = Unbundle By Name(w611) -> ("local data directory"=w616:path, "Data Save"=w604:refnum<class "Data.lvclass">)
        n236 = Path To String(path=w616) -> (string=w601:string)
        n237 = call <userlib>:"Tick Count (ms)__ogtk.vi"("error in (no error)"=w606) -> ("error out"=w591:errorcluster, "millisecond timer value"=w608:u32)  [unwired: 9 in]
        n238 = Concatenate Strings(w601, ".tdms") -> (w599:string)
        n239 = String To Path(string=w599) -> (path=w592:path)
        n240 = call "Read Unparsed Metadata from TDMS.vi"("error in (no error)"=w591, "file path"=w592) -> ("error out"=w589:errorcluster)  [unwired: 7 in, 2 out]
        n241 = call <userlib>:"Data Read.vi"("Append Index"=-1, "error in (no error)"=w589, "path"=w592) -> ("error out"=w598:errorcluster, "Notes"=→"Notes":string, "Data (Dictionary)"=w594:T11[])  [unwired: 5 in, 1 out]
        n242 = call <userlib>:"Write Data (Dictionary).vi"("error in (no error)"=w598, "Data (Dictionary)"=w594, "Data Save"=w604) -> ("error out"=w596:errorcluster, "Data Save out"=w597:refnum<class "Data.lvclass">)  [unwired: 7 in]
        n243 = call <userlib>:"Read Wavenames.vi"("error in (no error)"=w596, "Data Save"=w597) -> ("error out"=w586:errorcluster, "Wavenames"=w603:string[], "Data Save out"=w587:refnum<class "Data.lvclass">)  [unwired: 7 in]
        n244 = call "TDMS Get Number of Groups.vi"("error in (no error)"=w586, "path"=w592) -> ("error out"=w590:errorcluster, "# of groups"=w593:i32)  [unwired: 8 in]
        n245 = call "get data dimensions.vi"("# of groups"=w593, "Data (Dictionary)"=w594) -> ("data dimensions"=w602:i32[])  [unwired: 8 in, 1 out]
        "data dimensions" <- w602
        n246 = call <userlib>:"Tick Count (ms)__ogtk.vi"("error in (no error)"=w590) -> ("error out"=w605:errorcluster, "millisecond timer value"=w609:u32)  [unwired: 9 in]
        n247 = Bundle By Name(cluster=w611, "Data Save"=w587, "wavenames"=w603, "data dimensions"=w602) -> (w610:T8)
        n248 = Subtract(x=w609, y=w608) -> (x-y=→"cache load (ms)":u32)
        n249 = property on="reading cache" class="Bool (strict)"(error in=w605, "Value"=FALSE ("read cache")) -> (error out=w613:errorcluster)  [unwired: 1 in, 1 out]
        n250 = call <vilib>:"Add State(s) to Queue__jki_lib_state_machine.vi"("State(s) in (\"\")"=w618) -> ("States Out"=w617:string)  [unwired: 14 in]
      }
      frame "Load: Load from ITX" {
        # "Template Separator\n(You can make a copy of, or modify, this frame)"
        n251 = Unbundle By Name(w627) -> ("local data directory"=w626:path)
        n252 = call <userlib>:"Tick Count (ms)__ogtk.vi"("error in (no error)"=w625) -> ("error out"=w624:errorcluster, "millisecond timer value"=w620:u32)  [unwired: 9 in]
        n253 = call "open_itxFolder_to_labview.vi"("error in (no error)"=w624, "experiment folder (containing itx)"=w626) -> ("error out"=w623:errorcluster)  [unwired: 8 in, 1 out]
        n254 = disable-structure shown="Disabled" {
          disable-tunnel: [w632 w633] -> w628
          disable-tunnel: w627 -> [w631 w633]
          frame Disabled {
            n255 = Bundle By Name(cluster=w631) -> (w632:T8)  [unwired: 1 in]
          }
          frame Enabled {
          }
        }
        n256 = call <userlib>:"Tick Count (ms)__ogtk.vi"("error in (no error)"=w623) -> ("error out"=w622:errorcluster, "millisecond timer value"=w621:u32)  [unwired: 9 in]
        n257 = Subtract(x=w621, y=w620) -> (x-y=→"itx load (ms)":u32)
        n258 = call <vilib>:"Add State(s) to Queue__jki_lib_state_machine.vi"("State(s) in (\"\")"=w630) -> ("States Out"=w629:string)  [unwired: 14 in]
      }
      frame "Load: Populate Local Folder Tree" {
        # "Template Separator\n(You can make a copy of, or modify, this frame)"
        n259 = Unbundle By Name(w634) -> ("local data directory"=w639:path)
        n260 = List Folder(path=w639) -> (path out=w638:path, folder names=w637:string[])  [unwired: 3 in, 2 out]
        n261 = call-poly <userlib>:"Build Path__ogtk.vi"("name or relative path"=w637, "base path"=w638) -> ("appended path"=w635:path[])
        n262 = control-ref of="Local Tree"() -> (w640:refnum<vi>)
        n263 = invoke class="Tree (strict)" method="Edit Tree Items.Delete"(reference=w640, error in=w636) -> (reference out=w643:refnum<vi>, error out=w642:errorcluster)  [unwired: 3 in, 3 out]
        n264 = Path To String(path=w635) -> (string=w644:string[])
        n265 = for {
          tunnel: w643 -> [w648]
          tunnel: w644 -> [w647] mode=indexing
          shift-right: [w649] -> w641
          shift-left: w642 -> [w650]
          n266 = call "recursively populate local tree ctl.vi"("error in (no error)"=w650, "Object path"=w647, "tree ctl ref"=w648) -> ("error out"=w649:errorcluster)  [unwired: 7 in, 1 out]
        }
        n267 = call <vilib>:"Add State(s) to Queue__jki_lib_state_machine.vi"("State(s) in (\"\")"=w646) -> ("States Out"=w645:string)  [unwired: 14 in]
      }
    }
  }
  n268 = disable-structure shown="Disabled" {
    frame Disabled {
    }
    frame Enabled {
    }
  }
